vi "ajustePos.vi"(7 "dif Z":dbl=-8.0, 9 "p 50nm":dbl=100.0 format="%#_13g", 10 "p 100nm":dbl=1000.0 format="%#_13g", 11 "p 1000nm":dbl=3000.0 format="%#_13g") -> (2 "Paso":dbl=5.0)   [LabVIEW 2018]
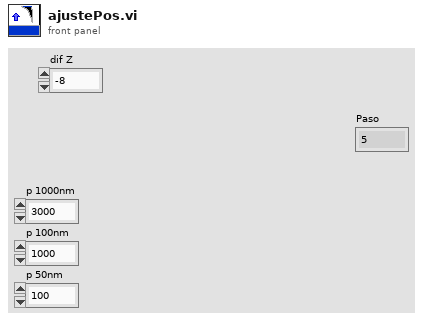
[diagram p1: front panel]
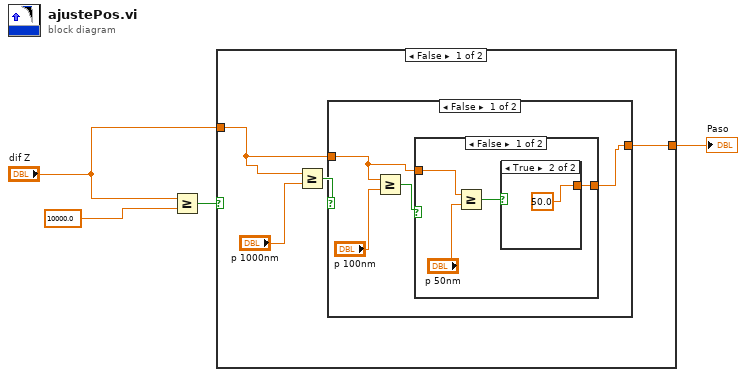
[diagram p0: block diagram]
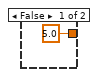
[diagram p2: hidden frame]
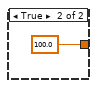
[diagram p3: hidden frame]
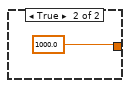
[diagram p4: hidden frame]
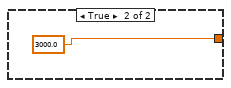
[diagram p5: hidden frame]
diagram:
  n1 = Greater Or Equal?(x="dif Z", y=10000.0) -> (x >= y?=w4:bool)
  n2 = case shown="False" w4 {
    tunnel: "dif Z" -> [w5 _]
    tunnel: [w6 3000.0] -> w1
    frame False {
      n3 = Greater Or Equal?(x=w5, y="p 1000nm") -> (x >= y?=w7:bool)
      n4 = case shown="False" w7 {
        tunnel: [w11 1000.0] -> w6
        tunnel: w5 -> [w9 _]
        frame False {
          n5 = Greater Or Equal?(x=w9, y="p 100nm") -> (x >= y?=w10:bool)
          n6 = case shown="False" w10 {
            tunnel: [w13 100.0] -> w11
            tunnel: w9 -> [w16 _]
            frame False {
              n7 = Greater Or Equal?(x=w16, y="p 50nm") -> (x >= y?=w14:bool)
              n8 = case shown="True" w14 {
                tunnel: [5.0 50.0] -> w13
                frame False {
                }
                frame True {
                }
              }
            }
            frame True {
            }
          }
        }
        frame True {
        }
      }
    }
    frame True {
    }
  }
  "Paso" <- w1
